vi "hello.vi"(8 "error in (no error)":errorcluster, 11 "Input":string) -> (0 "error out":errorcluster, 3 "Output":string)   [LabVIEW 2014]
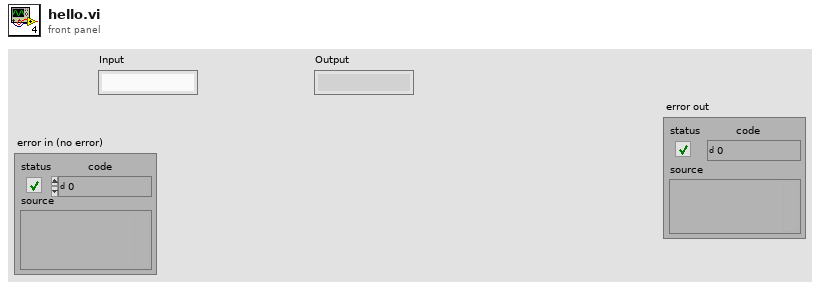
[diagram p1: front panel]
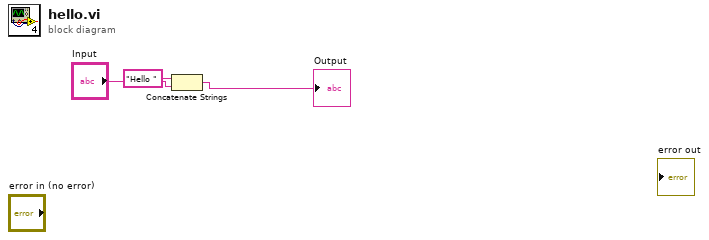
[diagram p0: block diagram]
diagram:
  n1 = Concatenate Strings("Hello " ("string"), "Input") -> (→"Output":string)
